vi "Create long wfm.vi"() -> ()   [LabVIEW 2019]
uses:
  <vilib>/Analysis/1siggen.llb/Ramp Pattern by Samples.vi
  <vilib>/Analysis/1siggen.llb/General Periodic Sinc.vi
  <vilib>/measure/matone.llb/Extract Single Tone Information 1 Chan.vi
  <vilib>/Analysis/NI_AALBase.lvlib
  <vilib>/measure/NI_MAPro.lvlib
panel:
  in  "cycles":dbl=10.0
  out "detected frequency":dbl format="%.2p"
  out "size(s)":i32
  out "signal":waveform(dbl)(graph)
  in  "sampling info":cluster{"Fs":dbl, "#s":dbl}={"Fs"=3072000000.0, "#s"=160000.0}
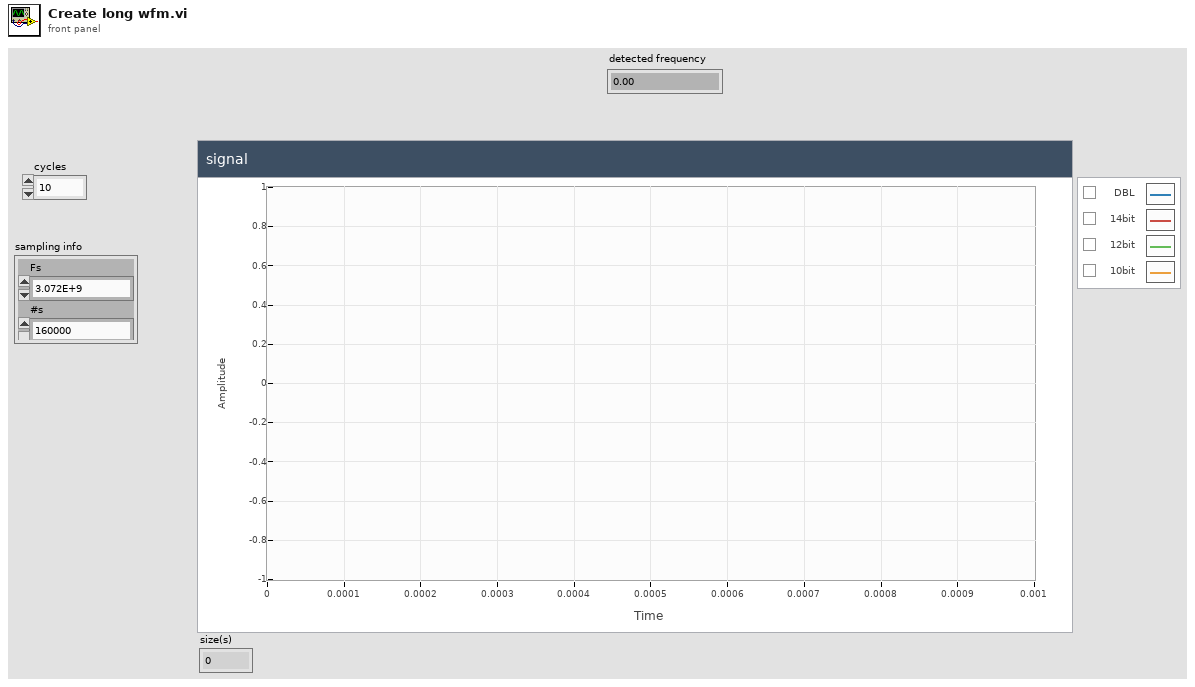
[diagram p1: front panel]
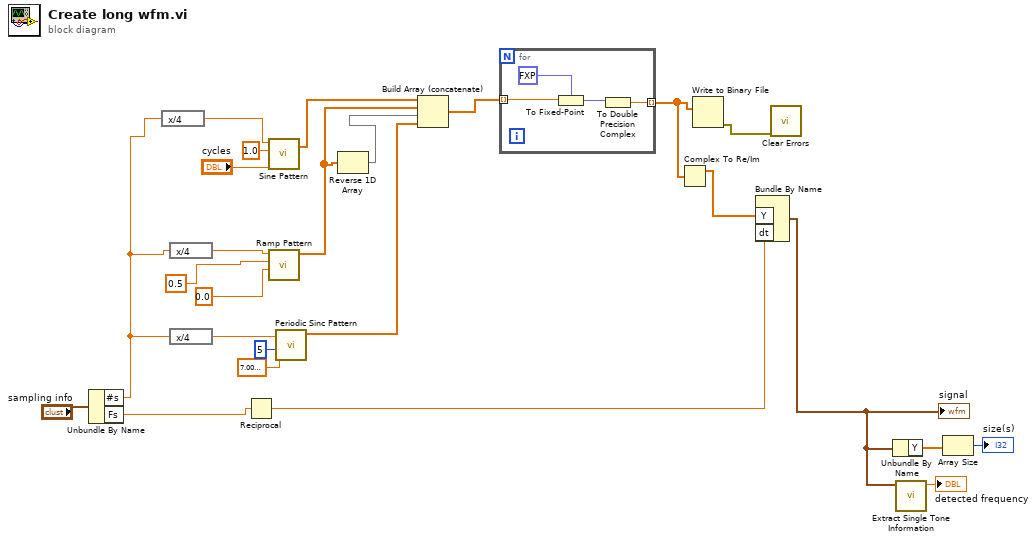
[diagram p0: block diagram]
diagram:
  n1 = Unbundle By Name("sampling info") -> ("#s"=w6:dbl, "Fs"=w22:dbl)
  n2 = expression code="x/4"(w6) -> (w12:dbl)
  n3 = expression code="x/4"(w6) -> (w11:dbl)
  n4 = expression code="x/4"(w6) -> (w5:dbl)
  n5 = Reciprocal(x=w22) -> (1/x=w2:dbl)
  n6 = call <vilib>:"Sine Pattern.vi"("cycles"="cycles", "amplitude"=1.0, "samples"=w12) -> ("Sinusoidal Pattern"=w17:dbl[])  [unwired: 1 in, 1 out]
  n7 = call-poly <vilib>:"Ramp Pattern.vi"("start"=0.0, "end"=0.5 ("start"), "samples"=w11) -> ("Ramp Pattern"=w8:dbl[])  [unwired: 7 in, 1 out]
  n8 = call <vilib>:"Periodic Sinc Pattern.vi"("delta t (s)"=7.000000000000001e-05, "order"=5, "samples"=w5) -> ("Periodic Sinc Pattern"=w4:dbl[])  [unwired: 7 in, 1 out]
  n9 = Reverse 1D Array(array=w8) -> (reversed array=w7:dbl[])
  n10 = Build Array (concatenate)(w17, w8, w7, w4) -> (w13:dbl[])
  n11 = for {
    tunnel: w13 -> [w29] mode=indexing
    tunnel: [w26] -> w15 mode=indexing
    n12 = To Fixed-Point(fixed-point type=fxp<+/-,14,1> 0.0, number=w29) -> (fixed-point=w27:fxp<+/-,14,1>)
    n13 = To Double Precision Complex(1:w27) -> (0:w26:cdb)
  }
  n14 = Complex To Re/Im(x + iy=w15) -> (x=w14:dbl[])  [unwired: 1 out]
  n15 = Write to Binary File(data=w15) -> (error out=w16:errorcluster)  [unwired: 5 in, 2 out]
  n16 = Bundle By Name("Y"=w14, "dt"=w2) -> (w20:waveform(dbl))  [unwired: 1 in]
  "signal" <- w20
  n17 = call <vilib>:"Clear Errors.vi"("error in (no error)"=w16) -> ()  [unwired: 5 in, 2 out]
  n18 = Unbundle By Name(w20) -> ("Y"=w21:dbl[])
  n19 = call-poly <vilib>:"Extract Single Tone Information.vi"("time signal in"=w20) -> ("detected frequency"=→"detected frequency":dbl)  [unwired: 5 in, 5 out]
  n20 = Array Size(array=w21) -> (size(s)=→"size(s)":i32)
